vi "Main.vi"() -> ()   [LabVIEW 2015]
uses:
  class/Car.lvclass
panel:
  in  "Obstacles":i32[][](array[numeric])
  in  "Scaling":dbl
  out "Instructions":i32[][](array[numeric])
  in  "Destinations":i32[][](array[numeric])
  in  "Start Y":i32=2
  in  "Start X":i32=2
  out "appended array":dbl[][](array[numeric])
  in  "Obstacles":bool[][](array[boolean])=[[TRUE, TRUE, TRUE, TRUE, TRUE, TRUE, TRUE, TRUE, TRUE, TRUE, TRUE, TRUE, TRUE, TRUE, TRUE, TRUE, TRUE, TRUE, TRUE], [TRUE, FALSE, FALSE, FALSE, FALSE, TRUE, FALSE, FALSE, FALSE, FALSE, FALSE, FALSE, FALSE, FALSE, FALSE, FALSE, FALSE, FALSE, TRUE], [TRUE, FALSE, FALSE, FALSE, FALSE, TRUE, FALSE, FALSE, FALSE, FALSE, FALSE, FALSE, FALSE, FALSE, FALSE, FALSE, FALSE, FALSE, TRUE], [TRUE, FALSE, FALSE, FALSE, FALSE, TRUE, FALSE, FALSE, FALSE, FALSE, TRUE, TRUE, TRUE, TRUE, TRUE, TRUE, FALSE, FALSE, TRUE], [TRUE, FALSE, FALSE, FALSE, FALSE, TRUE, FALSE, FALSE, FALSE, FALSE, TRUE, FALSE, FALSE, FALSE, FALSE, TRUE, FALSE, FALSE, TRUE], [TRUE, FALSE, FALSE, FALSE, FALSE, TRUE, FALSE, FALSE, FALSE, FALSE, TRUE, FALSE, FALSE, FALSE, FALSE, FALSE, FALSE, FALSE, TRUE], [TRUE, FALSE, FALSE, FALSE, FALSE, TRUE, FALSE, FALSE, FALSE, FALSE, TRUE, FALSE, FALSE, FALSE, FALSE, FALSE, FALSE, FALSE, TRUE], [TRUE, FALSE, FALSE, FALSE, FALSE, TRUE, FALSE, FALSE, FALSE, FALSE, TRUE, FALSE, FALSE, FALSE, FALSE, TRUE, FALSE, FALSE, TRUE], [TRUE, FALSE, FALSE, FALSE, FALSE, FALSE, FALSE, FALSE, FALSE, FALSE, TRUE, TRUE, TRUE, TRUE, TRUE, TRUE, FALSE, FALSE, TRUE], [TRUE, FALSE, FALSE, FALSE, FALSE, FALSE, FALSE, FALSE, FALSE, FALSE, FALSE, FALSE, FALSE, FALSE, FALSE, FALSE, FALSE, FALSE, TRUE], [TRUE, FALSE, FALSE, FALSE, FALSE, FALSE, FALSE, FALSE, FALSE, FALSE, FALSE, FALSE, FALSE, FALSE, FALSE, FALSE, FALSE, FALSE, TRUE], [TRUE, FALSE, FALSE, FALSE, FALSE, TRUE, FALSE, FALSE, FALSE, FALSE, FALSE, FALSE, FALSE, FALSE, FALSE, FALSE, FALSE, FALSE, TRUE], [TRUE, FALSE, FALSE, FALSE, FALSE, TRUE, FALSE, FALSE, FALSE, FALSE, FALSE, FALSE, FALSE, TRUE, FALSE, FALSE, FALSE, FALSE, TRUE], [TRUE, FALSE, FALSE, FALSE, FALSE, TRUE, FALSE, FALSE, FALSE, FALSE, FALSE, FALSE, FALSE, TRUE, FALSE, FALSE, FALSE, FALSE, TRUE], [TRUE, TRUE, TRUE, TRUE, TRUE, TRUE, TRUE, TRUE, TRUE, TRUE, TRUE, TRUE, TRUE, TRUE, TRUE, TRUE, TRUE, TRUE, TRUE]]
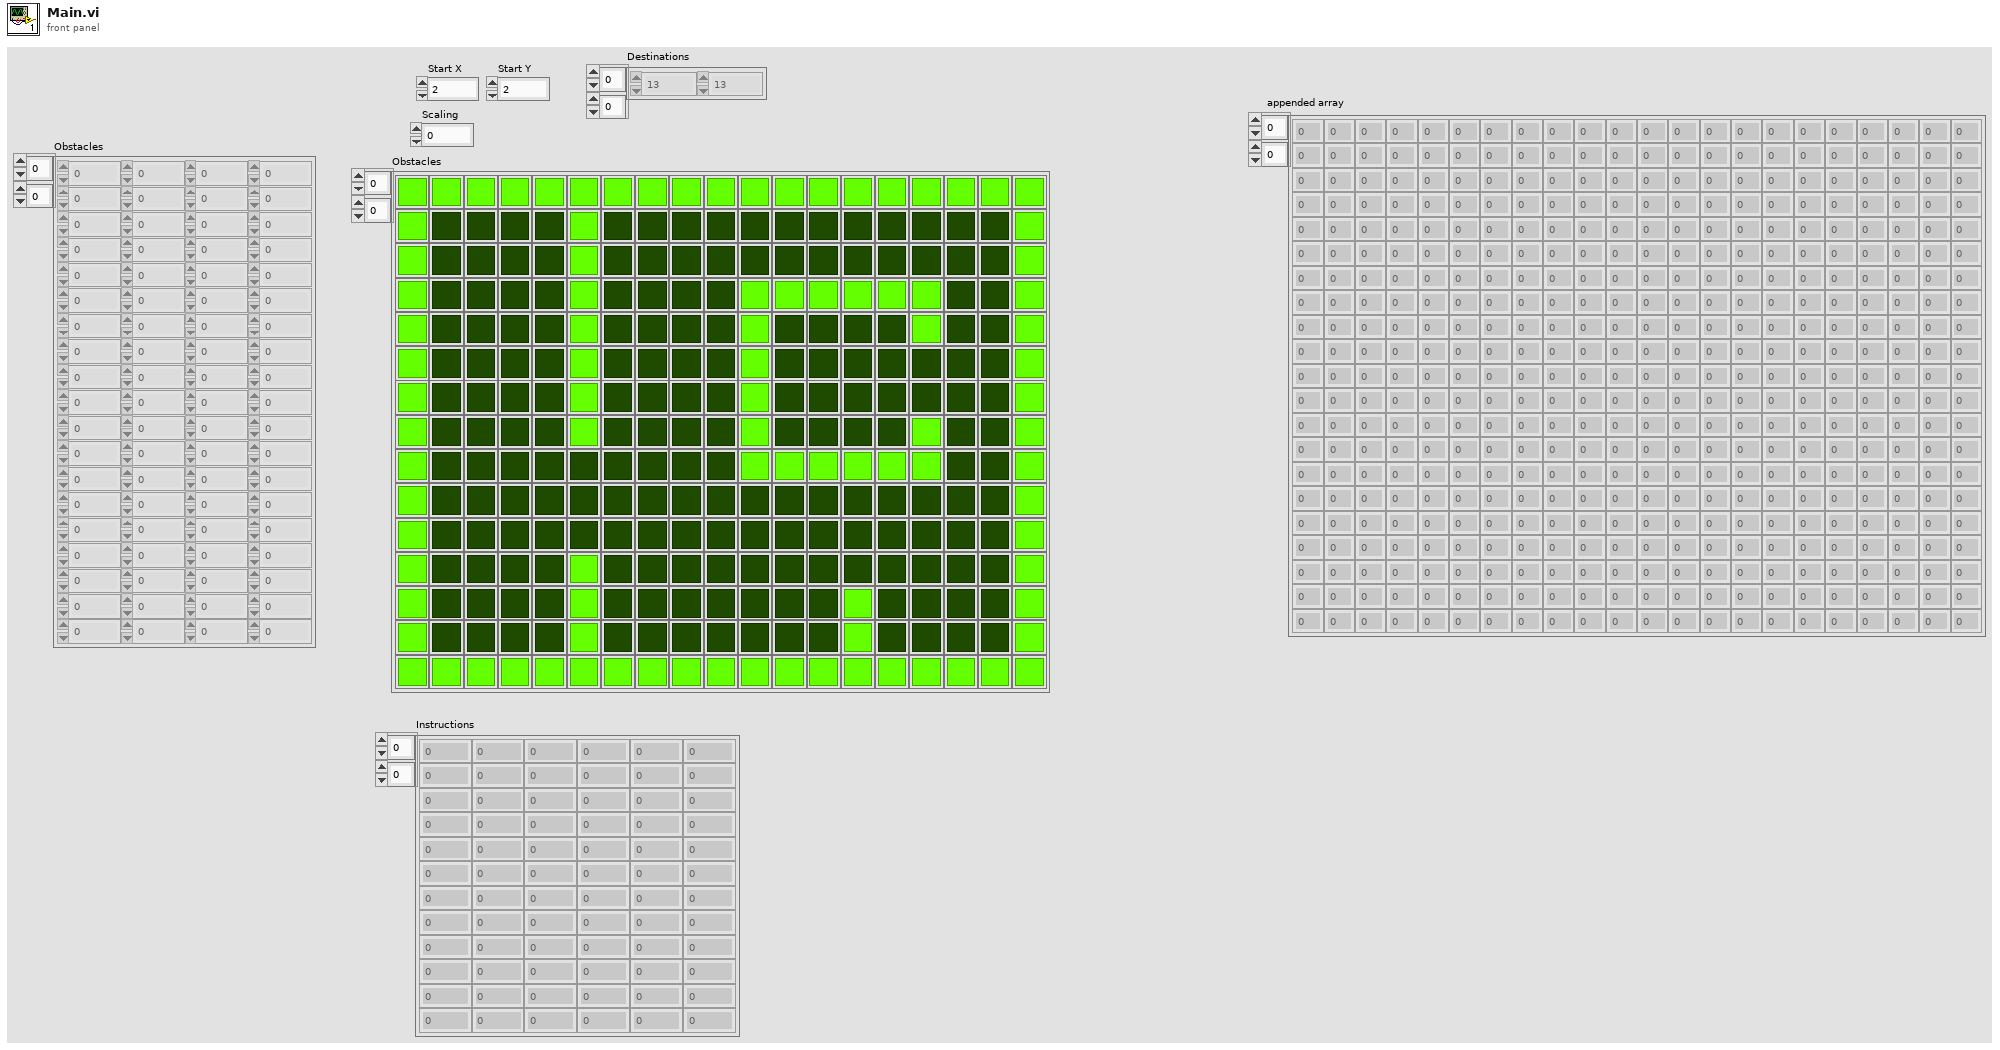
[diagram p1: front panel]
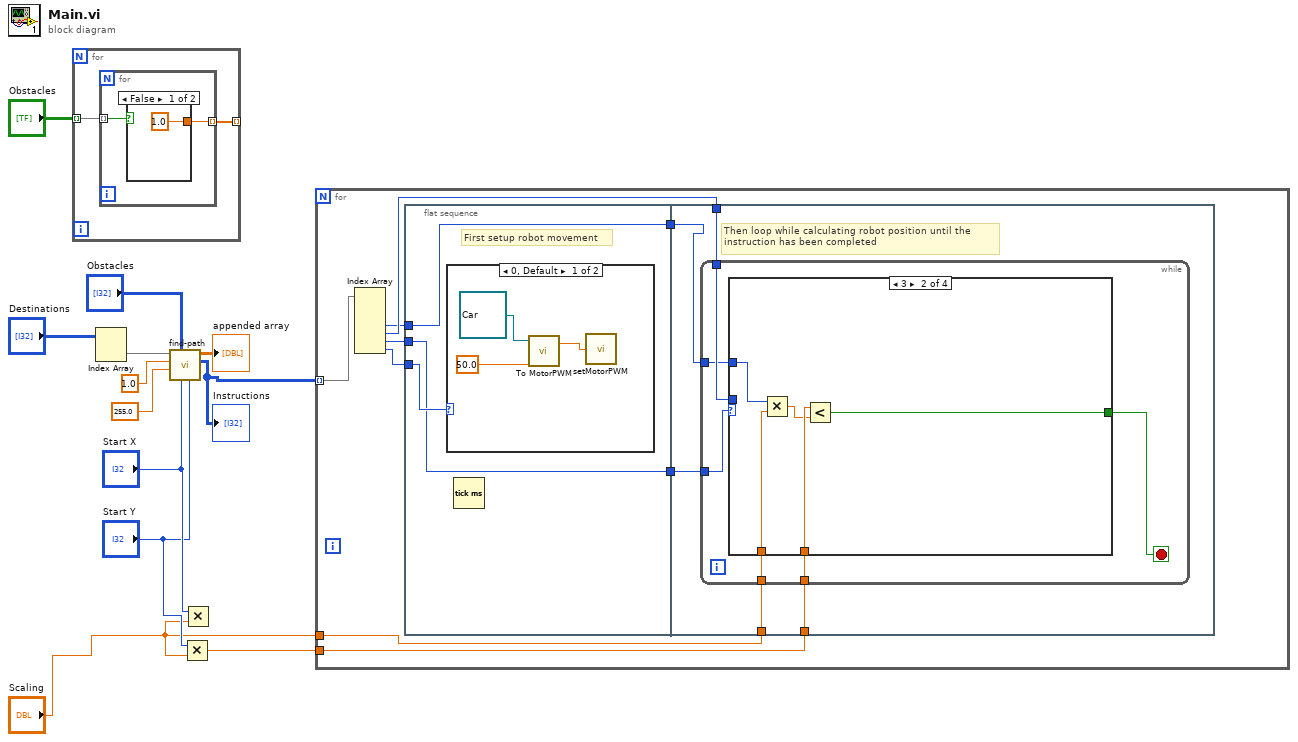
[diagram p0: block diagram]
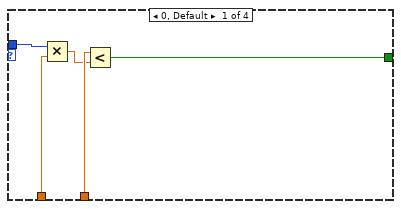
[diagram p3: hidden frame]
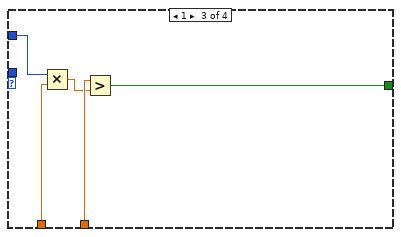
[diagram p4: hidden frame]
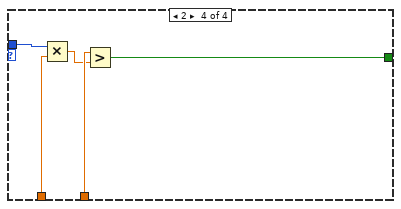
[diagram p5: hidden frame]
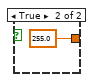
[diagram p6: hidden frame]
diagram:
  n1 = for {
    tunnel: "Obstacles" -> [w14] mode=indexing
    tunnel: [w13] -> _ mode=indexing
    n2 = for {
      tunnel: w14 -> [w16] mode=indexing
      tunnel: [w15] -> w13 mode=indexing
      n3 = case shown="False" w16 {
        tunnel: [1.0 255.0] -> w15
        frame False {
        }
        frame True {
        }
      }
    }
  }
  n4 = Index Array(array="Destinations") -> (element=w6:i32[])  [unwired: 2 in]
  n5 = call "find-path.vi"("Start Y"="Start Y", "Start X"="Start X", "Obstacles"="Obstacles", "Numeric"=255.0, "Numeric 2"=1.0, "Destination"=w6) -> ("Instructions"=w5:i32[][], "appended array"=→"appended array":dbl[][])  [unwired: 4 in]
  "Instructions" <- w5
  n6 = Multiply(x="Start Y", y="Scaling") -> (x*y=w2:dbl)
  n7 = Multiply(x="Start X", y="Scaling") -> ()  [unwired: 1 out]
  n8 = for {
    tunnel: w5 -> [w27] mode=indexing
    tunnel: w2 -> [w23]
    tunnel: "Scaling" -> [w22]
    n9 = Index Array(array=w27) -> (element #3=w19:i32, element #4=w21:i32, element #5=w25:i32, element #6=w26:i32)  [unwired: 6 in, 2 out]
    n10 = flat-sequence {
      tunnel: w26 -> [w30]
      tunnel: w25 -> [w29]
      tunnel: [w29] -> w24
      tunnel: [w28] -> w20
      tunnel: w19 -> [w28]
      tunnel: w24 -> [w38]
      tunnel: w23 -> [w37]
      tunnel: w22 -> [w36]
      tunnel: w21 -> [w35]
      tunnel: w20 -> [w34]
      frame #0 {
        # "First setup robot movement"
        n11 = case shown="0, Default" w30 {
          frame 0, Default {
            n12 = call "To MotorPWM.vi"("Speed"=50.0, "Car.lvclass"=refnum<class "Car.lvclass"> refnum) -> ("MotorPWM"=w32:dbl)  [unwired: 1 in, 1 out]
            n13 = call "setMotorPWM.vi"("Numeric"=w32) -> ()
          }
          frame 1 {
          }
        }
        n14 = Tick Count (ms)() -> ()  [unwired: 1 out]
      }
      frame #1 {
        # "Then loop while calculating robot position until the \ninstruction has been completed"
        n15 = while {
          tunnel: w38 -> [w44]
          tunnel: w37 -> [w43]
          tunnel: w36 -> [w42]
          tunnel: w35 -> [w41]
          tunnel: w34 -> [w39]
          stop <- w40 stop-if-true
          n16 = case shown="3" w44 {
            tunnel: w43 -> [w49 w54 w59 w64]
            tunnel: w42 -> [w47 w52 w57 w62]
            tunnel: w41 -> [w46 _ _ w61]
            tunnel: [w45 w51 w56 w60] -> w40
            tunnel: w39 -> [_ w50 w55 _]
            frame 0, Default {
              n17 = Multiply(x=w46, y=w47) -> (x*y=w48:dbl)
              n18 = Less?(x=w49, y=w48) -> (x < y?=w45:bool)
            }
            frame 3 {
              n19 = Multiply(x=w50, y=w52) -> (x*y=w53:dbl)
              n20 = Less?(x=w54, y=w53) -> (x < y?=w51:bool)
            }
            frame 1 {
              n21 = Multiply(x=w55, y=w57) -> (x*y=w58:dbl)
              n22 = Greater?(x=w59, y=w58) -> (0:w56:bool)
            }
            frame 2 {
              n23 = Multiply(x=w61, y=w62) -> (x*y=w63:dbl)
              n24 = Greater?(x=w64, y=w63) -> (0:w60:bool)
            }
          }
        }
      }
    }
  }
